vi "Build GUI List.vi"(8 "error in (no error)":errorcluster, 11 "GUI Manager Module in":refnum<class "GUI Manager Module.lvclass">) -> (0 "error out":errorcluster, 2 "GUIs":T1[](array[typedef]), 3 "GUI Manager Module out":refnum<class "GUI Manager Module.lvclass">)   [LabVIEW 2020, in "VolatusGUI.lvlib" / "GUI Manager Module.lvclass"]
uses:
  GUI Manager Module.lvclass
  GUI Manager Module.lvclass/GUI Manager Module.ctl
  GUI Entry.ctl
  68ee1954-2421-4577-9498-3e8168589279.vi
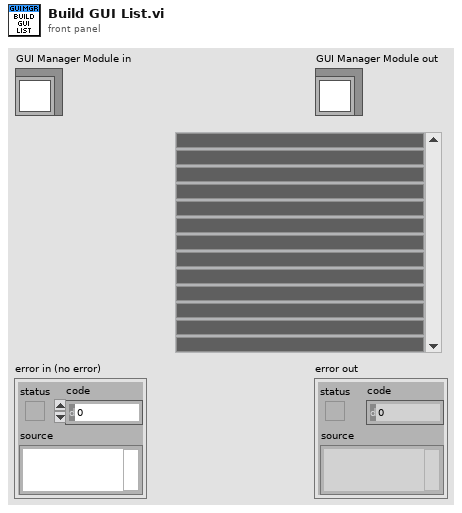
[diagram p1: front panel]
types:
  T1 = typedef "VolatusGUI.lvlib/GUI Manager Module.lvclass/GUI Entry.ctl" = cluster{"Name Color":u32, "Name":string, "Show GUI":bool, "ID":string}
  T2 = typedef "VolatusGUI.lvlib/GUI Registration.ctl" = cluster{"ID":string, "GUI Helper":refnum<class "MessageQ.lvclass">, "Module":refnum<class "MessageQ.lvclass">, "Info":T3, "Open":bool}
  T3 = typedef "VolatusGUI.lvlib/GUI Info.ctl" = cluster{"Color":u32, "Name":string}
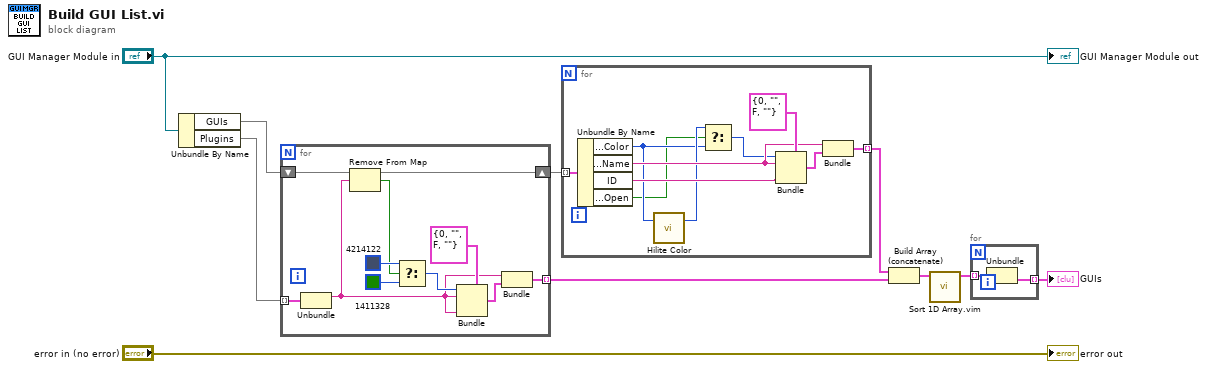
[diagram p0: block diagram]
diagram:
  n1 = Unbundle By Name("GUI Manager Module in") -> ("GUIs"=w7:map{string, T2}, "Plugins"=w8:map{string, path})
  n2 = for {
    tunnel: w8 -> [w21] mode=indexing
    tunnel: [w12] -> w5 mode=indexing
    shift-right: [w15] -> w6
    shift-left: w7 -> [w19]
    n3 = Unbundle(w21) -> (w11:string)  [unwired: 1 out]
    n4 = Remove From Map(10:w11, 11:w19) -> (2:w16:bool, 3:w15:map{string, T2})  [unwired: 1 out]
    n5 = Select(t=u32 4214122, s=w16, f=u32 1411328) -> (s? t:f=w14:u32)
    n6 = Bundle(cluster=T1 {"Name Color"=0, "Name"="", "Show GUI"=FALSE, "ID"=""} ("GUI Entry"), "Name Color"=w14, "Name"=w11, "ID"=w11) -> (w13:T1)  [unwired: 1 in]
    n7 = Bundle(w11, "GUI Entry"=w13) -> (w12:cluster{string, "GUI Entry":T1})  [unwired: 1 in]
  }
  n8 = for {
    tunnel: w6 -> [w28] mode=indexing
    tunnel: [w29] -> w4 mode=indexing
    n9 = Unbundle By Name(w28) -> ("GUI Registration.Info.Color"=w24:u32, "GUI Registration.Info.Name"=w27:string, "ID"=w26:string, "GUI Registration.Open"=w22:bool)
    n10 = call <vilib>:"Hilite Color.vi"("Color In"=w24) -> ("Hilite"=w25:u32)  [unwired: 1 in, 1 out]
    n11 = Select(t=w25, s=w22, f=w24) -> (s? t:f=w23:u32)
    n12 = Bundle(cluster=T1 {"Name Color"=0, "Name"="", "Show GUI"=FALSE, "ID"=""} ("GUI Entry"), "Name Color"=w23, "Name"=w27, "ID"=w26) -> (w30:T1)  [unwired: 1 in]
    n13 = Bundle("Name"=w27, "GUI Entry"=w30) -> (w29:cluster{"Name":string, "GUI Entry":T1})  [unwired: 1 in]
  }
  n14 = Build Array (concatenate)(w4, w5) -> (w3:cluster{"Name":string, "GUI Entry":T1}[])
  n15 = call "Sort 1D Array.vim"("unsorted array"=w3) -> ("sorted array"=w2:cluster{"Name":string, "GUI Entry":T1}[])  [unwired: 10 in]
  n16 = for {
    tunnel: w2 -> [w33] mode=indexing
    tunnel: [w32] -> w1 mode=indexing
    n17 = Unbundle(w33) -> ("GUI Entry"=w32:T1)  [unwired: 1 out]
  }
  "GUIs" <- w1
  "error out" <- "error in (no error)"
  "GUI Manager Module out" <- "GUI Manager Module in"
